vi "SDG60ConfModulationAM.vi"(5 "Depth (100.0%)":dbl=100.0 format="%#_16g", 6 "Frequency (1.0 Hz)":dbl=1.0 format="%#_16g", 7 "Mod wave shape (0:Sine)":u16(ring) items=["Sine", "Square", "Triangle", "Up Ramp", "Down Ramp", "Noise", "Arb"], 8 "error in (no error)":errorcluster, 9 "Internal/External (0: INT)":u16(ring) items=["Internal", "External", "Ch1", "Ch2"], 10 "Channel (1:Channel 1)":i32(ring)=1 items=["Channel 1"=1, "Channel 2"=2], 11 "VISA resource name":refnum<visa-resource-name>="USB0::0xF4EC::0x1101::SDG6XEBC5R0119::INSTR") -> (0 "error out":errorcluster, 3 "VISA resource name out":refnum<visa-resource-name>)   [LabVIEW 2018]
doc: "Selects the waveform shape, frequency, amplitude, offset, and phase for standard waveforms (including Sine, Square, Ramp, Pulse, DC and Arb).\n\nNotes: \nTo configure other parameters for pulse waveforms please run the Configure Pulse VI. \nTo configure noise waveform please run the Configure Noise VI.\nTo configure other parameters for arbitrary waveforms please run the Create Arbitrary Waveform. \nTo configure PRBS waveform please run the Configure PRBS Waveform VI."
panel:
  in  "State(T:On)":bool=TRUE
  # "Can set WFM then use this vi. No need to setup carrier.\nModulation can't be done on noise, DC (Not testing IQ as has trials)\nSet modulaton after setting up carrier WFM!"
  # "Modulation will be turned on, as needed to be on to change\nsettings. Done through SDG60ModulationOnOff vi\nCan't suppres the carrier spectral component effectively by changing the depth\n\nMode shape, freq, depth not changable when set to external"
  # "With external, +/-5.5V is needed for full sweep modulation. For Ch1 and Ch2 the modulating channel needs to have ouptput in ON state, can only be activated via virtual keys - unreliable don't use\nstate for modulation to work"
  # "ARB can only be chosen from front panel. Noise doesn't give 100% depth even at 120% setting."
  # "Range: 0.001Hz-1 MHz\n11 digit precision"
  # "Range: 0-120%\n11 digit precision"
  # "Depth=Am/Ac where Am is amp (not Pk-Pk!) of modulated signal, Ac is amp of carrier \nDepth=(Amax-Amin)/(Amax+Amin) where Amax/Amin are max/min amp of modulated wave"
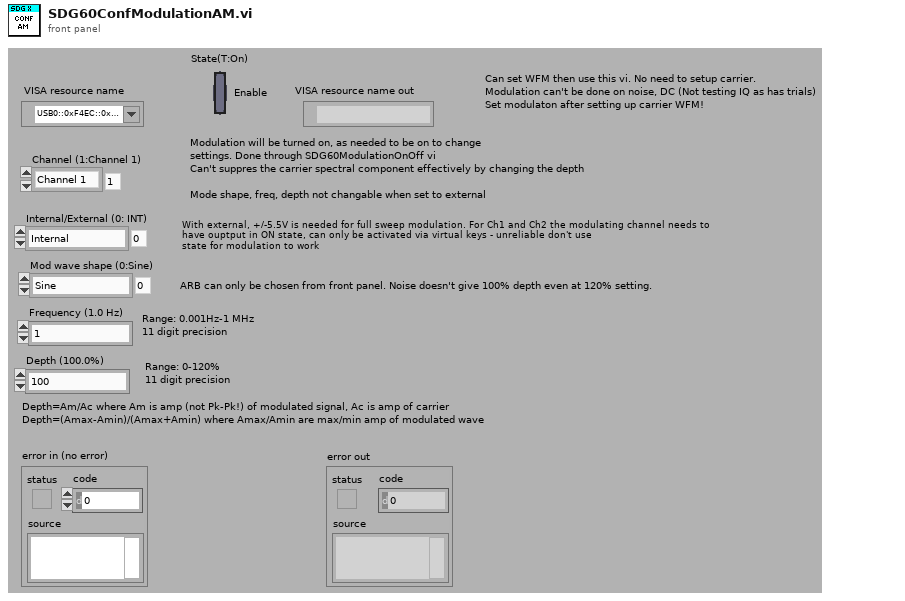
[diagram p1: front panel]
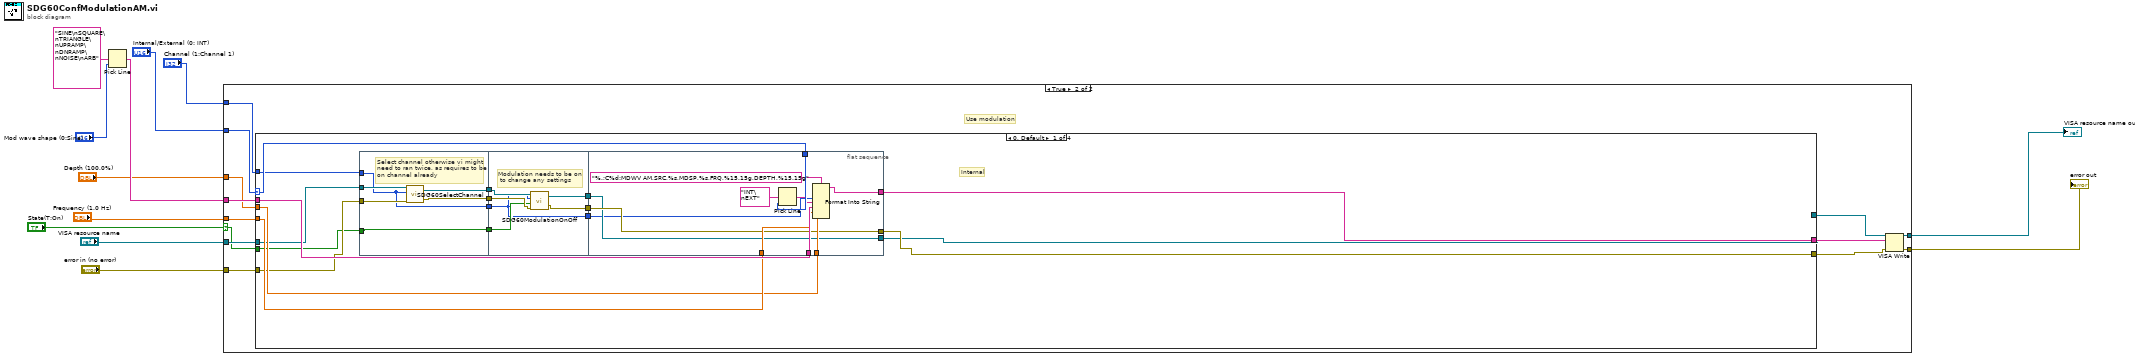
[diagram p0: block diagram]
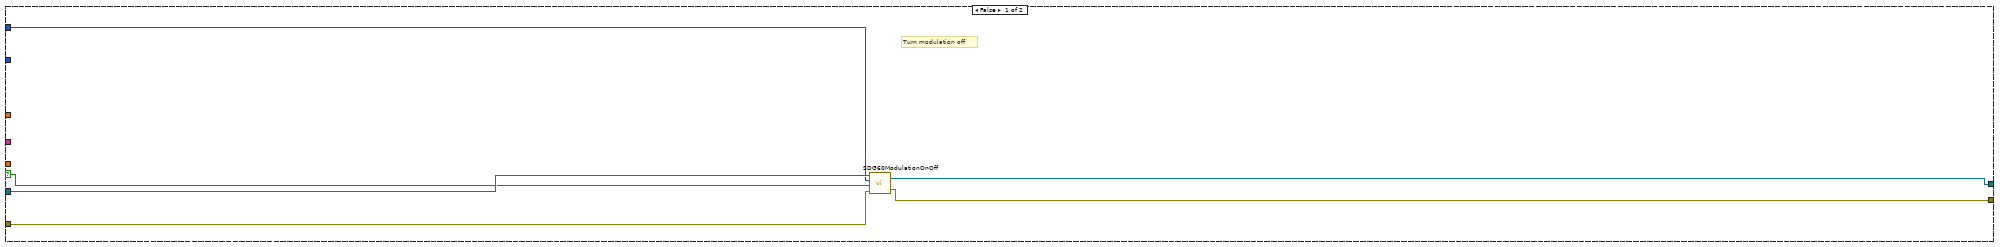
[diagram p2: hidden frame]
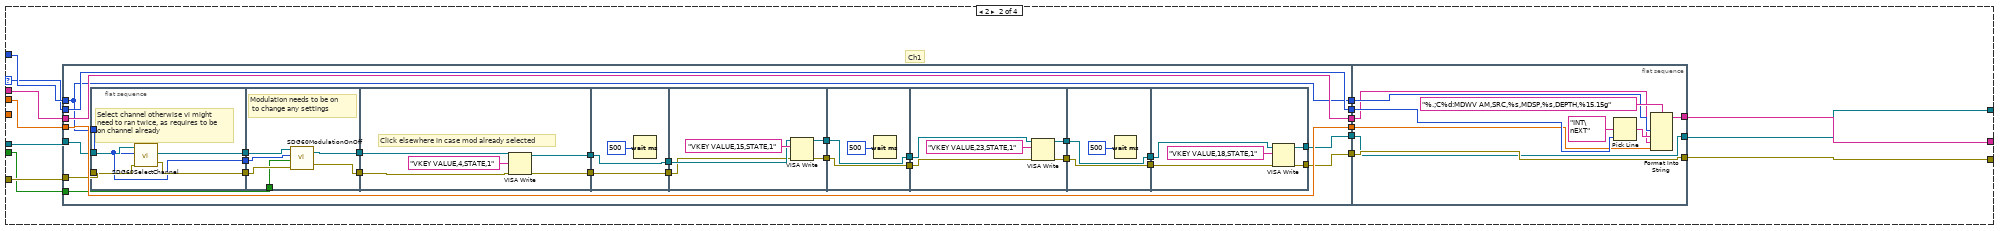
[diagram p3: hidden frame]
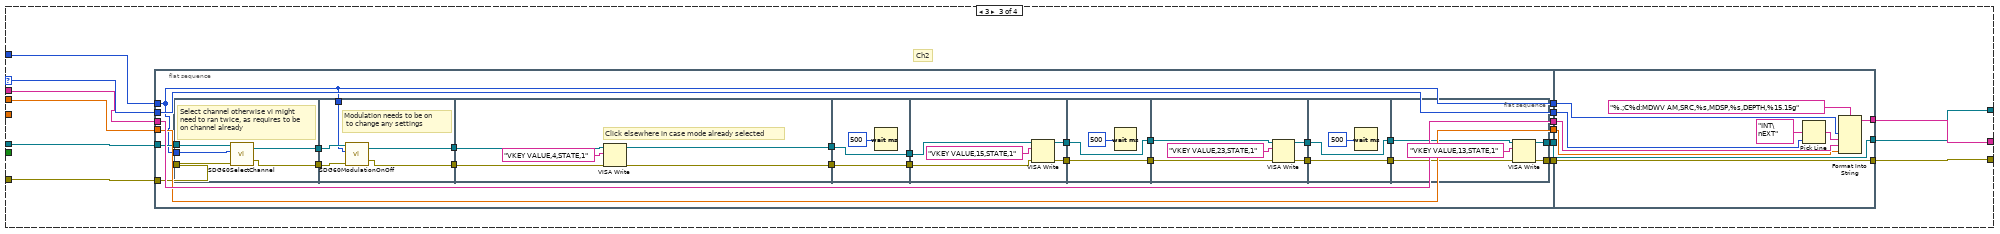
[diagram p4: hidden frame]
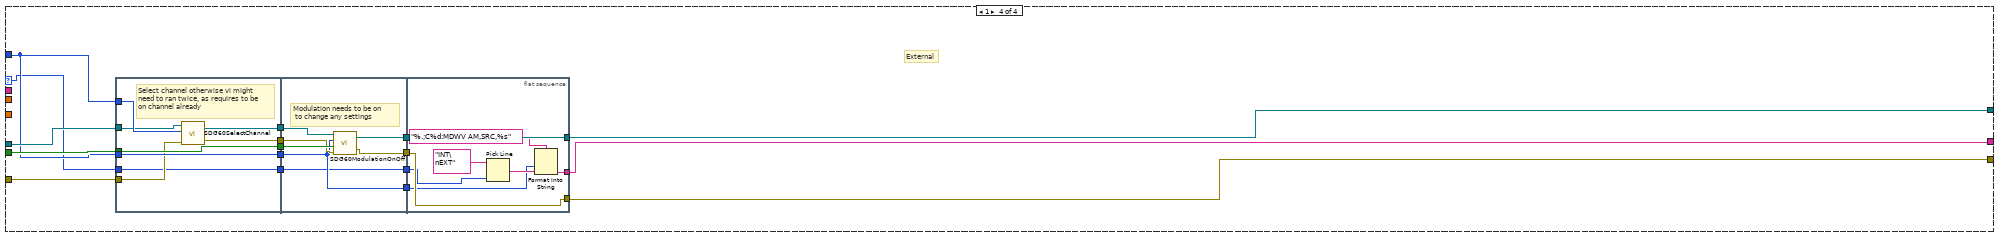
[diagram p5: hidden frame]
diagram:
  n1 = Pick Line(multi-line string="SINE\nSQUARE\nTRIANGLE\nUPRAMP\nDNRAMP\nNOISE\nARB", line index="Mod wave shape (0:Sine)") -> (output string=w6:string)  [unwired: 1 in]
  n2 = case shown="True" "State(T:On)" {
    selector: "State(T:On)" -> [w15 w19]
    tunnel: [w14 w30] -> w12
    tunnel: [w13 w29] -> w11
    tunnel: "Channel (1:Channel 1)" -> [w16 w28]
    tunnel: "Internal/External (0: INT)" -> [_ w27]
    tunnel: w6 -> [_ w26]
    tunnel: "Frequency (1.0 Hz)" -> [_ w25]
    tunnel: "Depth (100.0%)" -> [_ w24]
    tunnel: "error in (no error)" -> [w17 w23]
    tunnel: "VISA resource name" -> [w18 w22]
    frame False {
      # "Turn modulation off"
      n3 = call "SDG60ModulationOnOff.vi"("error in (no error)"=w17, "Enable Output (T: Enable)"=w15, "Channel (1: Channel1)"=w16, "VISA resource name"=w18) -> ("error out"=w13:errorcluster, "VISA resource name out"=w14:refnum<visa-resource-name>)
    }
    frame True {
      # "Use modulation"
      n4 = case shown="0, Default" w27 {
        selector: w27 -> [w46 w86 w177 w255]
        tunnel: [w42 w88 w179 w269] -> w31
        tunnel: w28 -> [w36 w87 w178 w257]
        tunnel: w26 -> [w45 w85 w176 _]
        tunnel: w25 -> [w44 _ _ _]
        tunnel: w24 -> [w43 w84 w175 _]
        tunnel: w22 -> [w37 w79 w170 w263]
        tunnel: w23 -> [w41 w78 w169 w258]
        tunnel: [w40 w76 w167 w268] -> w20
        tunnel: [w39 w74 w165 w267] -> w21
        tunnel: w19 -> [w34 w73 _ w261]
        frame 0, Default {
          # "Internal"
          n5 = flat-sequence {
            tunnel: [w55] -> w49
            tunnel: w41 -> [w54]
            tunnel: [w53] -> w38
            tunnel: w37 -> [w52]
            tunnel: w36 -> [w50]
            tunnel: w34 -> [w51]
            tunnel: [w51] -> w35
            tunnel: [w50] -> w33
            tunnel: [w61] -> w48
            tunnel: [w60] -> w47
            tunnel: w49 -> [w59]
            tunnel: w38 -> [w58]
            tunnel: w35 -> [w57]
            tunnel: w33 -> [w56]
            tunnel: [w56] -> w32
            tunnel: w48 -> [w66]
            tunnel: w47 -> [w65]
            tunnel: w46 -> [w72]
            tunnel: w45 -> [w70]
            tunnel: w44 -> [w69]
            tunnel: w43 -> [w68]
            tunnel: [w67] -> w42
            tunnel: [w66] -> w40
            tunnel: [w65] -> w39
            tunnel: w32 -> [w64]
            frame #0 {
              # "Select channel otherwise vi might \nneed to ran twice, as requires to be\non channel already"
              n6 = call "SDG60SelectChannel.vi"("error in (no error)"=w54, "Channel (1: Channel1)"=w50, "VISA resource name"=w52) -> ("error out"=w55:errorcluster, "VISA resource name out"=w53:refnum<visa-resource-name>)  [unwired: 1 in]
            }
            frame #1 {
              # "Modulation needs to be on\n to change any settings"
              n7 = call "SDG60ModulationOnOff.vi"("error in (no error)"=w59, "Enable Output (T: Enable)"=w57, "Channel (1: Channel1)"=w56, "VISA resource name"=w58) -> ("error out"=w61:errorcluster, "VISA resource name out"=w60:refnum<visa-resource-name>)
            }
            frame #2 {
              n8 = Pick Line(multi-line string="INT\nEXT", line index=w72) -> (output string=w62:string)  [unwired: 1 in]
              n9 = Format Into String(format string="%.;C%d:MDWV AM,SRC,%s,MDSP,%s,FRQ,%15.15g,DEPTH,%15.15g", w64, w62, w70, w69, w68) -> (resulting string=w67:string)  [unwired: 2 in, 1 out]
            }
          }
        }
        frame 2 {
          # "Ch1"
          n10 = flat-sequence {
            tunnel: w84 -> [w112]
            tunnel: w85 -> [w113]
            tunnel: w86 -> [w114]
            tunnel: w87 -> [w95]
            tunnel: [w95] -> w83
            tunnel: [w114] -> w82
            tunnel: [w113] -> w81
            tunnel: [w112] -> w80
            tunnel: w79 -> [w107]
            tunnel: w78 -> [w106]
            tunnel: [w105] -> w77
            tunnel: [w104] -> w75
            tunnel: w73 -> [w90]
            tunnel: [w163] -> w88
            tunnel: w83 -> [w162]
            tunnel: w82 -> [w161]
            tunnel: w81 -> [w158]
            tunnel: w80 -> [w157]
            tunnel: w77 -> [w156]
            tunnel: [w156] -> w76
            tunnel: [w155] -> w74
            tunnel: w75 -> [w155]
            frame #0 {
              n11 = flat-sequence {
                tunnel: w106 -> [w117]
                tunnel: w107 -> [w118]
                tunnel: [w119] -> w94
                tunnel: [w116] -> w92
                tunnel: w95 -> [w115]
                tunnel: [w115] -> w89
                tunnel: w94 -> [w125]
                tunnel: [w124] -> w93
                tunnel: w92 -> [w122]
                tunnel: [w123] -> w91
                tunnel: w90 -> [w121]
                tunnel: w89 -> [w120]
                tunnel: [w129] -> w111
                tunnel: [w127] -> w110
                tunnel: w93 -> [w130]
                tunnel: w91 -> [w126]
                tunnel: w111 -> [w133]
                tunnel: [w133] -> w109
                tunnel: [w131] -> w108
                tunnel: w110 -> [w131]
                tunnel: w109 -> [w137]
                tunnel: w108 -> [w134]
                tunnel: [w136] -> w103
                tunnel: [w135] -> w101
                tunnel: w103 -> [w141]
                tunnel: [w141] -> w102
                tunnel: w101 -> [w140]
                tunnel: [w140] -> w100
                tunnel: w102 -> [w146]
                tunnel: w100 -> [w144]
                tunnel: [w142] -> w99
                tunnel: [w143] -> w97
                tunnel: w99 -> [w149]
                tunnel: [w149] -> w98
                tunnel: w97 -> [w148]
                tunnel: [w148] -> w96
                tunnel: [w153] -> w105
                tunnel: [w154] -> w104
                tunnel: w98 -> [w151]
                tunnel: w96 -> [w152]
                frame #0 {
                  # "Select channel otherwise vi might \nneed to ran twice, as requires to be\non channel already"
                  n12 = call "SDG60SelectChannel.vi"("error in (no error)"=w117, "Channel (1: Channel1)"=w115, "VISA resource name"=w118) -> ("error out"=w116:errorcluster, "VISA resource name out"=w119:refnum<visa-resource-name>)  [unwired: 1 in]
                }
                frame #1 {
                  # "Modulation needs to be on\n to change any settings"
                  n13 = call "SDG60ModulationOnOff.vi"("error in (no error)"=w122, "Enable Output (T: Enable)"=w121, "Channel (1: Channel1)"=w120, "VISA resource name"=w125) -> ("error out"=w123:errorcluster, "VISA resource name out"=w124:refnum<visa-resource-name>)
                }
                frame #2 {
                  # "Click elsewhere in case mod already selected"
                  n14 = VISA Write(VISA resource name=w130, write buffer="VKEY VALUE,4,STATE,1", error in (no error)=w126) -> (VISA resource name out=w129:refnum<visa-resource-name>, error out=w127:errorcluster)  [unwired: 1 out]
                }
                frame #3 {
                  n15 = Wait (ms)(milliseconds to wait=500) -> ()  [unwired: 1 out]
                }
                frame #4 {
                  n16 = VISA Write(VISA resource name=w137, write buffer="VKEY VALUE,15,STATE,1", error in (no error)=w134) -> (VISA resource name out=w136:refnum<visa-resource-name>, error out=w135:errorcluster)  [unwired: 1 out]
                }
                frame #5 {
                  n17 = Wait (ms)(milliseconds to wait=500) -> ()  [unwired: 1 out]
                }
                frame #6 {
                  n18 = VISA Write(VISA resource name=w146, write buffer="VKEY VALUE,23,STATE,1", error in (no error)=w144) -> (VISA resource name out=w142:refnum<visa-resource-name>, error out=w143:errorcluster)  [unwired: 1 out]
                }
                frame #7 {
                  n19 = Wait (ms)(milliseconds to wait=500) -> ()  [unwired: 1 out]
                }
                frame #8 {
                  n20 = VISA Write(VISA resource name=w151, write buffer="VKEY VALUE,18,STATE,1", error in (no error)=w152) -> (VISA resource name out=w154:refnum<visa-resource-name>, error out=w153:errorcluster)  [unwired: 1 out]
                }
              }
            }
            frame #1 {
              n21 = Pick Line(multi-line string="INT\nEXT", line index=w161) -> (output string=w159:string)  [unwired: 1 in]
              n22 = Format Into String(format string="%.;C%d:MDWV AM,SRC,%s,MDSP,%s,DEPTH,%15.15g", w162, w159, w158, w157) -> (resulting string=w163:string)  [unwired: 2 in, 1 out]
            }
          }
        }
        frame 3 {
          # "Ch2"
          n23 = flat-sequence {
            tunnel: w175 -> [w201]
            tunnel: w176 -> [w202]
            tunnel: w177 -> [w203]
            tunnel: w178 -> [w180]
            tunnel: [w180] -> w174
            tunnel: [w203] -> w173
            tunnel: [w202] -> w172
            tunnel: [w201] -> w171
            tunnel: w170 -> [w196]
            tunnel: w169 -> [w195]
            tunnel: [w194] -> w168
            tunnel: [w193] -> w166
            tunnel: [w251] -> w179
            tunnel: w174 -> [w250]
            tunnel: w173 -> [w249]
            tunnel: w172 -> [w246]
            tunnel: w171 -> [w245]
            tunnel: w168 -> [w244]
            tunnel: [w244] -> w167
            tunnel: [w243] -> w165
            tunnel: w166 -> [w243]
            frame #0 {
              n24 = flat-sequence {
                tunnel: w195 -> [w205]
                tunnel: w196 -> [w208]
                tunnel: [w207] -> w184
                tunnel: [w206] -> w183
                tunnel: w180 -> [w204]
                tunnel: w184 -> [w213]
                tunnel: w183 -> [w210]
                tunnel: [w211] -> w182
                tunnel: [w212] -> w181
                tunnel: w180 -> [w209]
                tunnel: [w217] -> w200
                tunnel: [w215] -> w199
                tunnel: w182 -> [w214]
                tunnel: w181 -> [w218]
                tunnel: w200 -> [w221]
                tunnel: [w221] -> w198
                tunnel: [w219] -> w197
                tunnel: w199 -> [w219]
                tunnel: w198 -> [w225]
                tunnel: w197 -> [w222]
                tunnel: [w224] -> w192
                tunnel: [w223] -> w190
                tunnel: w192 -> [w229]
                tunnel: [w229] -> w191
                tunnel: w190 -> [w228]
                tunnel: [w228] -> w189
                tunnel: w191 -> [w234]
                tunnel: w189 -> [w232]
                tunnel: [w230] -> w188
                tunnel: [w231] -> w186
                tunnel: w188 -> [w237]
                tunnel: [w237] -> w187
                tunnel: w186 -> [w236]
                tunnel: [w236] -> w185
                tunnel: [w241] -> w194
                tunnel: [w242] -> w193
                tunnel: w187 -> [w239]
                tunnel: w185 -> [w240]
                frame #0 {
                  # "Select channel otherwise vi might \nneed to ran twice, as requires to be\non channel already"
                  n25 = call "SDG60SelectChannel.vi"("error in (no error)"=w205, "Channel (1: Channel1)"=w204, "VISA resource name"=w208) -> ("error out"=w206:errorcluster, "VISA resource name out"=w207:refnum<visa-resource-name>)  [unwired: 1 in]
                }
                frame #1 {
                  # "Modulation needs to be on\n to change any settings"
                  n26 = call "SDG60ModulationOnOff.vi"("error in (no error)"=w210, "Channel (1: Channel1)"=w209, "VISA resource name"=w213) -> ("error out"=w211:errorcluster, "VISA resource name out"=w212:refnum<visa-resource-name>)  [unwired: 1 in]
                }
                frame #2 {
                  # "Click elsewhere in case mode already selected"
                  n27 = VISA Write(VISA resource name=w218, write buffer="VKEY VALUE,4,STATE,1", error in (no error)=w214) -> (VISA resource name out=w217:refnum<visa-resource-name>, error out=w215:errorcluster)  [unwired: 1 out]
                }
                frame #3 {
                  n28 = Wait (ms)(milliseconds to wait=500) -> ()  [unwired: 1 out]
                }
                frame #4 {
                  n29 = VISA Write(VISA resource name=w225, write buffer="VKEY VALUE,15,STATE,1", error in (no error)=w222) -> (VISA resource name out=w224:refnum<visa-resource-name>, error out=w223:errorcluster)  [unwired: 1 out]
                }
                frame #5 {
                  n30 = Wait (ms)(milliseconds to wait=500) -> ()  [unwired: 1 out]
                }
                frame #6 {
                  n31 = VISA Write(VISA resource name=w234, write buffer="VKEY VALUE,23,STATE,1", error in (no error)=w232) -> (VISA resource name out=w230:refnum<visa-resource-name>, error out=w231:errorcluster)  [unwired: 1 out]
                }
                frame #7 {
                  n32 = Wait (ms)(milliseconds to wait=500) -> ()  [unwired: 1 out]
                }
                frame #8 {
                  n33 = VISA Write(VISA resource name=w239, write buffer="VKEY VALUE,13,STATE,1", error in (no error)=w240) -> (VISA resource name out=w242:refnum<visa-resource-name>, error out=w241:errorcluster)  [unwired: 1 out]
                }
              }
            }
            frame #1 {
              n34 = Pick Line(multi-line string="INT\nEXT", line index=w249) -> (output string=w247:string)  [unwired: 1 in]
              n35 = Format Into String(format string="%.;C%d:MDWV AM,SRC,%s,MDSP,%s,DEPTH,%15.15g", w250, w247, w246, w245) -> (resulting string=w251:string)  [unwired: 2 in, 1 out]
            }
          }
        }
        frame 1 {
          # "External"
          n36 = flat-sequence {
            tunnel: [w271] -> w264
            tunnel: w263 -> [w272]
            tunnel: w261 -> [w277]
            tunnel: [w277] -> w262
            tunnel: w257 -> [w276]
            tunnel: [w276] -> w260
            tunnel: [w275] -> w259
            tunnel: w258 -> [w274]
            tunnel: w257 -> [w273]
            tunnel: w255 -> [w270]
            tunnel: [w270] -> w253
            tunnel: [w284] -> w266
            tunnel: [w283] -> w265
            tunnel: w264 -> [w282]
            tunnel: w262 -> [w281]
            tunnel: w260 -> [w279]
            tunnel: w259 -> [w280]
            tunnel: [w279] -> w256
            tunnel: [w278] -> w254
            tunnel: w253 -> [w278]
            tunnel: [w291] -> w267
            tunnel: [w292] -> w268
            tunnel: [w287] -> w269
            tunnel: w266 -> [w292]
            tunnel: w265 -> [w291]
            tunnel: w256 -> [w286]
            tunnel: w254 -> [w285]
            frame #0 {
              # "Select channel otherwise vi might \nneed to ran twice, as requires to be\non channel already"
              n37 = call "SDG60SelectChannel.vi"("error in (no error)"=w274, "Channel (1: Channel1)"=w273, "VISA resource name"=w272) -> ("error out"=w275:errorcluster, "VISA resource name out"=w271:refnum<visa-resource-name>)  [unwired: 1 in]
            }
            frame #1 {
              # "Modulation needs to be on\n to change any settings"
              n38 = call "SDG60ModulationOnOff.vi"("error in (no error)"=w280, "Enable Output (T: Enable)"=w281, "Channel (1: Channel1)"=w279, "VISA resource name"=w282) -> ("error out"=w284:errorcluster, "VISA resource name out"=w283:refnum<visa-resource-name>)
            }
            frame #2 {
              n39 = Pick Line(multi-line string="INT\nEXT", line index=w285) -> (output string=w290:string)  [unwired: 1 in]
              n40 = Format Into String(format string="%.;C%d:MDWV AM,SRC,%s", w286, w290) -> (resulting string=w287:string)  [unwired: 2 in, 1 out]
            }
          }
        }
      }
      n41 = VISA Write(VISA resource name=w21, write buffer=w31, error in (no error)=w20) -> (VISA resource name out=w30:refnum<visa-resource-name>, error out=w29:errorcluster)  [unwired: 1 out]
    }
  }
  "error out" <- w11
  "VISA resource name out" <- w12
